vi "magnet_ps_pd_test.vi"(5 "STOP 2":bool, 7 "Mask":T1=16 items=["Flush Receive Buffer"=16, "Write Transmit Buffer to Device"=32, "Flush Receive Buffer (No I/O)"=64, "Flush Transmit Buffer"=128], 8 "error in":errorcluster, 10 "termination char\n(0xA = '\\n' = LF)":u8=10 format="%.0x", 11 "VISA resource name":refnum<visa-resource-name>="COM40") -> (0 "error out":errorcluster, 2 "Shim Coil 2":bool, 3 "Shim Coil 1":bool, 4 "read buffer":string)   [LabVIEW 2019]
uses:
  <vilib>/Instr/_visa.llb/VISA Flush IO Buffer Mask.ctl
panel:
  out "Background Intensity":i32(graph)=907
  # "Shim Coil 1"
  # "Shim Coil 2"
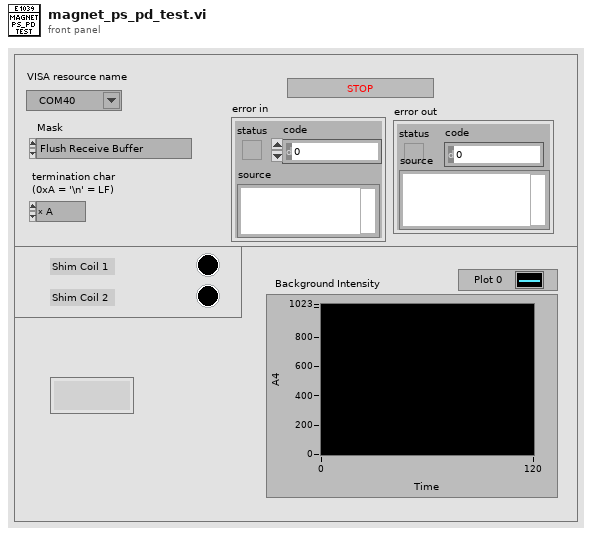
[diagram p1: front panel]
types:
  T1 = typedef "VISA Flush IO Buffer Mask.ctl" = u16
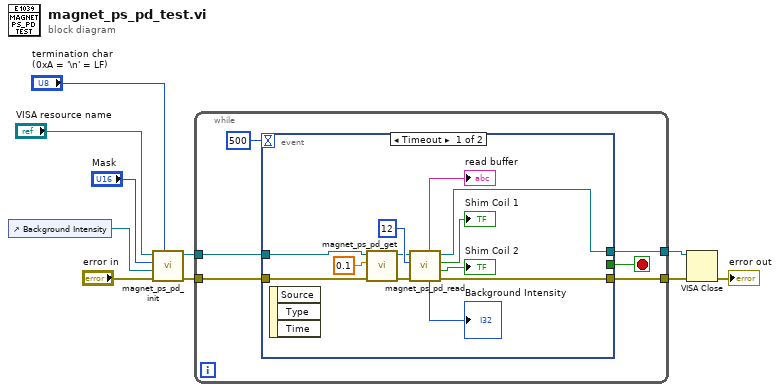
[diagram p0: block diagram]
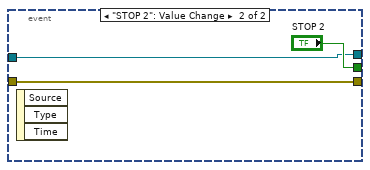
[diagram p2: hidden frame]
diagram:
  n1 = control-ref of="Background Intensity"() -> (w1:refnum<vi>)
  n2 = call "magnet_ps_pd_init.vi"("termination char\n(0xA = '\\n' = LF)"="termination char\n(0xA = '\\n' = LF)", "error in"="error in", "Chart reference"=w1, "Mask"="Mask", "VISA resource name"="VISA resource name") -> ("error out"=w2:errorcluster, "VISA resource name out"=w3:refnum<visa-resource-name>)  [unwired: 4 in, 1 out]
  n3 = while {
    tunnel: [w16] -> w9
    tunnel: w3 -> [w14]
    tunnel: [w15] -> w8
    tunnel: w2 -> [w11]
    stop <- w12 stop-if-true
    n4 = event shown="[0] Timeout" {
      selector: _ -> [_ _]
      dyn-events: _ -> [_ _]
      timeout: 500 -> [_ _]
      tunnel: [w20 w30] -> w16
      tunnel: [w21 w29] -> w15
      tunnel: w14 -> [w27 w30]
      tunnel: w11 -> [w28 w29]
      tunnel: [_ "STOP 2"] -> w12
      event Timeout {
        n5 = event-data() -> ()  [unwired: 1 in, 3 out]
        n6 = call "magnet_ps_pd_get.vi"("error in (no error)"=w28, "Wait untill read (S)"=0.1, "VISA resource name"=w27) -> ("error out"=w24:errorcluster, "VISA resource name out"=w23:refnum<visa-resource-name>)  [unwired: 7 in]
        n7 = call "magnet_ps_pd_read.vi"("error in (no error)"=w24, "byte count to read"=u32 12 ("byte count"), "VISA resource name"=w23) -> ("error out"=w21:errorcluster, "Shim Coil 2"=→"Shim Coil 2":bool, "Shim Coil 1"=→"Shim Coil 1":bool, "VISA resource name out"=w20:refnum<visa-resource-name>, "Background intensity (raw)"=→"Background Intensity":i32, "read buffer"=→"read buffer":string)  [unwired: 3 in]
      }
      event "STOP 2": Value Change {
        n8 = event-data() -> ()  [unwired: 1 in, 3 out]
      }
    }
  }
  n9 = VISA Close(VISA resource name=w9, error in (no error)=w8) -> (error out=→"error out":errorcluster)
